vi "A 侧面 处理函数CCD4.vi"(7 "Image Name":string="I1", 8 "error in (no error)":errorcluster caption="错误输入（无错误）", 9 "相机选择":T2="cam0" caption="Session Out CCD3", 10 "New Image":T1, 11 "ParamsUI":T3={"IsNorImage"=TRUE, "Exposure Values"=100289, "ImagePath"=path "C:/Users/hedongpo/Desktop/514-hdp/Alignment Assemble System/Test Picture/B/3.bmp", "相机选择"="cam4"} caption="参数界面" {"Exposure Values" scale=0.0..200000.0}) -> (0 "error out":errorcluster caption="错误输出", 2 "Session Out":T2, 3 "Image out":T1(plugin-control), 4 "数值":dbl)   [LabVIEW 2017]
uses:
  <vilib>/userdefined/High Color/IMAQdx.ctl
  <vilib>/vision/Image Controls.llb/IMAQ Image.ctl
  <vilib>/vision/driver/IMAQdx.llb/IMAQdx Buffer Number Mode.ctl
  <resource>/objmgr/imaqdx.rc
  Global System.vi
  <vilib>/vision/driver/NI_Vision_Acquisition_Software.lvlib
  <vilib>/vision/NI_Vision_Development_Module.lvlib
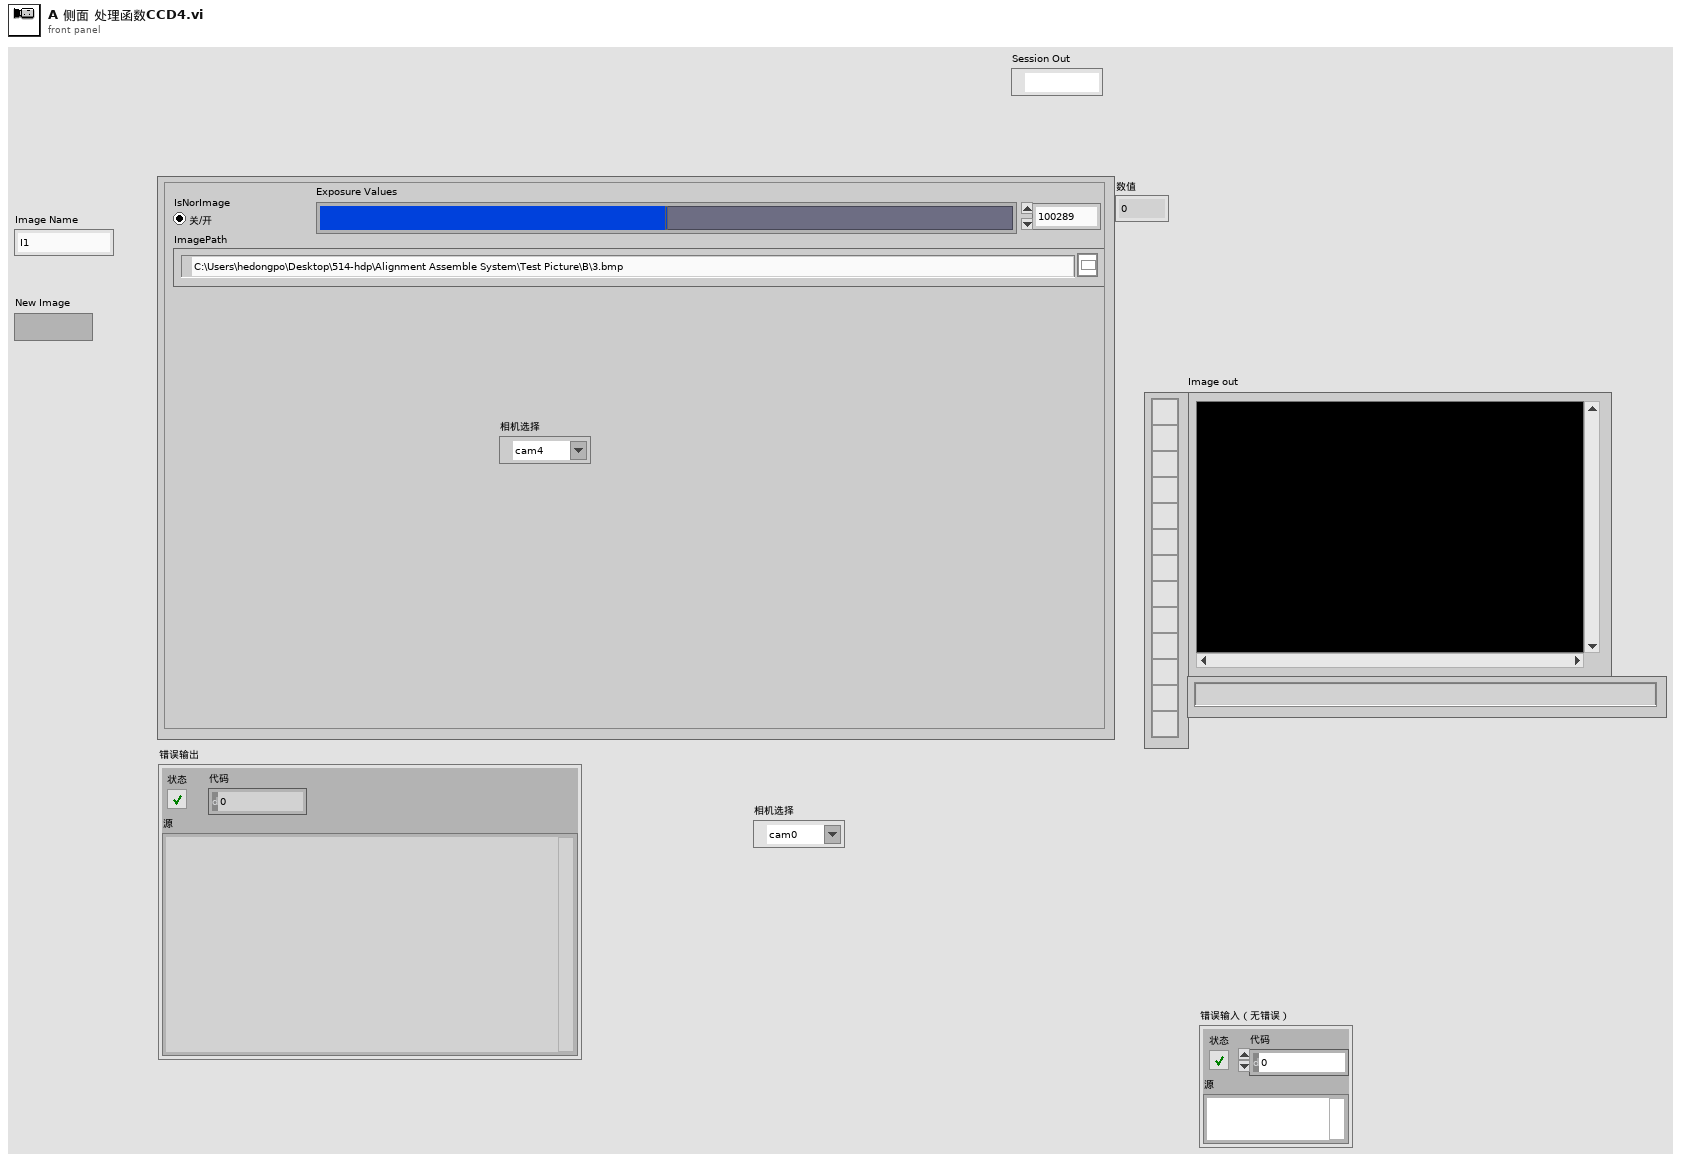
[diagram p1: front panel]
types:
  T1 = typedef "IMAQ Image.ctl" = refnum<image>
  T2 = typedef "IMAQdx.ctl" = refnum<k21>
  T3 = cluster{"IsNorImage":bool, "Exposure Values":i64, "ImagePath":path, "相机选择":T2}
  T4 = typedef "Image Type" = u32
  T5 = cluster{"IsNorImage":bool, "Exposure Values":u32, "ImagePath":path}
  T6 = typedef "NI_Vision_Acquisition_Software.lvlib/IMAQdx Buffer Number Mode.ctl" = enum32{"Next", "Last", "Buffer Number", "Every", "Last New"}
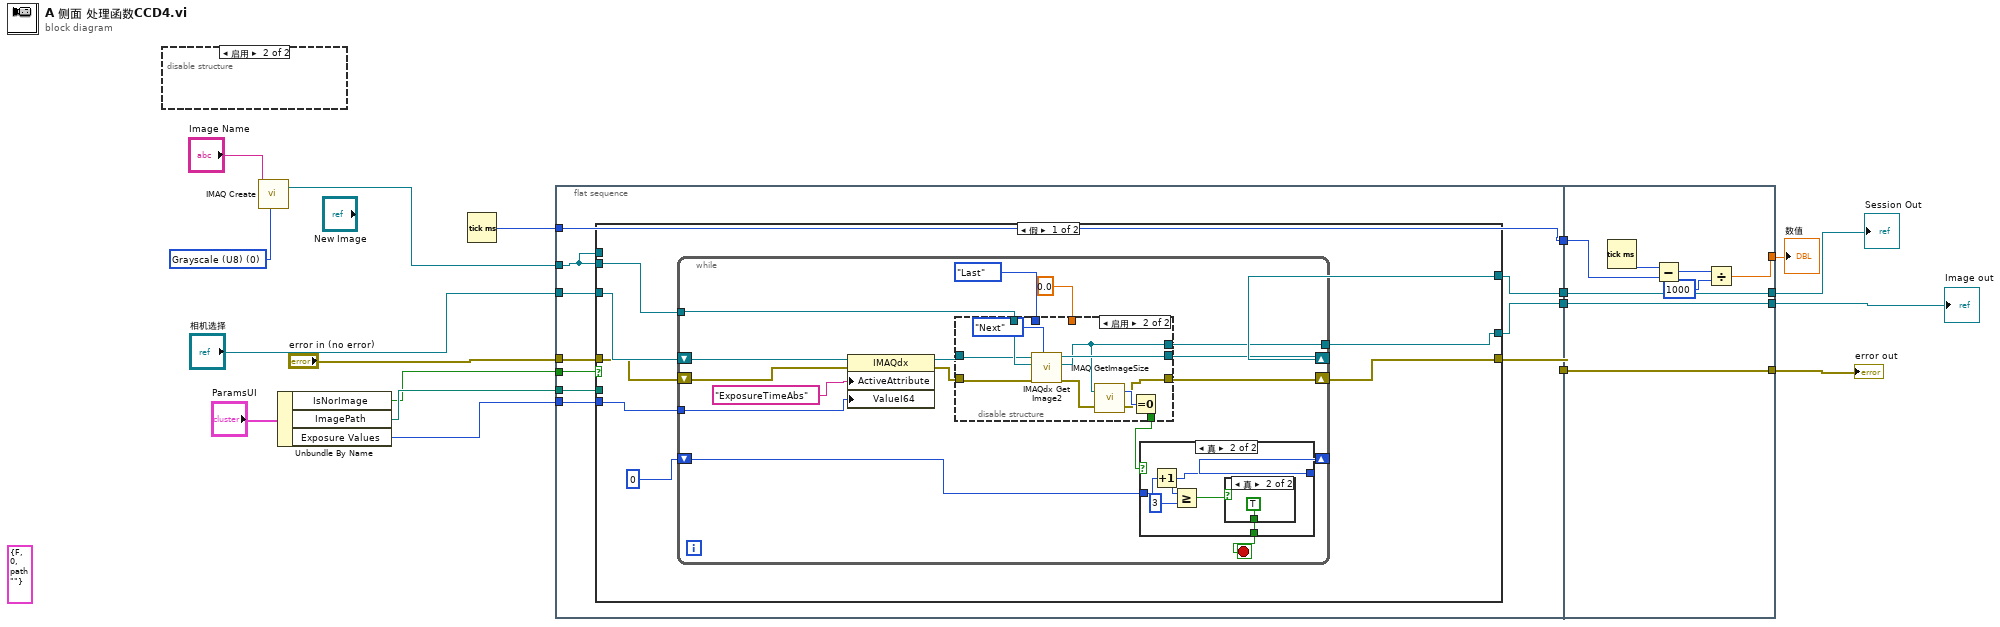
[diagram p0: block diagram]
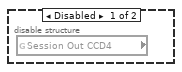
[diagram p2: hidden frame]
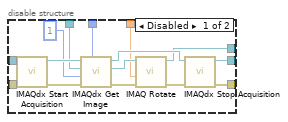
[diagram p3: hidden frame]
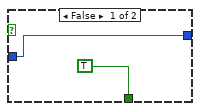
[diagram p4: hidden frame]
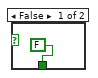
[diagram p5: hidden frame]
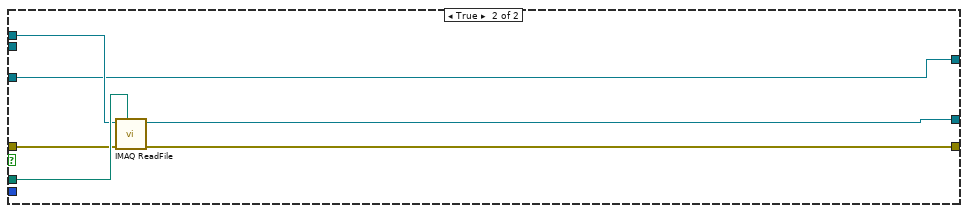
[diagram p6: hidden frame]
diagram:
  w2 = T4 0 items=["Grayscale (U8)", "Grayscale (I16)", "Grayscale (SGL)", "Complex (CSG)", "RGB (U32)", "HSL (U32)", "RGB (U64)", "Grayscale (U16)"] ("Image Type")
  (unwired) T5 {"IsNorImage"=FALSE, "Exposure Values"=0, "ImagePath"=path ""} ("ParamsUI")
  n1 = disable-structure shown="启用" {
    frame Disabled {
      n2 = global read "Global System.vi" "Session Out CCD4"() -> ()  [unwired: 1 out]
    }
    frame Enabled {
    }
  }
  n3 = call "IMAQ Create"("Image Name"="Image Name", "Image Type"=w2) -> ("New Image"=w1:T1)  [unwired: 3 in, 1 out]
  n4 = Unbundle By Name("ParamsUI") -> ("IsNorImage"=w5:bool, "ImagePath"=w6:path, "Exposure Values"=w18:i64)
  n5 = Tick Count (ms)() -> (millisecond timer value=w12:u32)
  n6 = flat-sequence {
    tunnel: w5 -> [w28]
    tunnel: w6 -> [w27]
    tunnel: w18 -> [w26]
    tunnel: w1 -> [w19]
    tunnel: "error in (no error)" -> [w25]
    tunnel: "相机选择" -> [w22]
    tunnel: w12 -> [w20]
    tunnel: [w24] -> w11
    tunnel: [w23] -> w10
    tunnel: [w21] -> w9
    tunnel: [w20] -> w8
    tunnel: [w98] -> w13
    tunnel: [w99] -> w14
    tunnel: [w100] -> w16
    tunnel: w11 -> [w100]
    tunnel: w10 -> [w99]
    tunnel: w9 -> [w98]
    tunnel: w8 -> [w96]
    tunnel: [w93] -> w7
    frame #0 {
      n7 = case shown="假" w28 {
        tunnel: w27 -> [_ w92]
        tunnel: [w29 w91] -> w23
        tunnel: w26 -> [w34 _]
        tunnel: w22 -> [w36 w87]
        tunnel: w19 -> [_ w90]
        tunnel: w25 -> [w35 w89]
        tunnel: [w30 w88] -> w24
        tunnel: [w31 w87] -> w21
        tunnel: w19 -> [w32 _]
        frame False {
          n8 = while {
            tunnel: w34 -> [w50]
            shift-right: [w39] -> w31
            shift-left: w36 -> [w52]
            shift-right: [w40] -> w30
            shift-left: w35 -> [w51]
            shift-right: [w47] -> _
            shift-left: 0 -> [w48]
            tunnel: w32 -> [w43]
            tunnel: [w38] -> w29
            stop <- w46 stop-if-true
            n9 = property class="IMAQdx"(reference=w52, error in=w51, "ActiveAttribute"="ExposureTimeAbs", "ValueI64"=w50) -> (reference out=w42:T2, error out=w41:errorcluster)
            n10 = disable-structure shown="启用" {
              disable-tunnel: IMAQdx_Buffer_Number_Mode."Last" ("Buffer Number Mode (Next)") -> [w64 _]
              disable-tunnel: sgl 0.0 ("Angle (degrees)") -> [w59 _]
              disable-tunnel: w43 -> [w58 w76]
              disable-tunnel: [w57 w73] -> w38
              disable-tunnel: [w56 w74] -> w39
              disable-tunnel: [w55 w69] -> w40
              disable-tunnel: w42 -> [w54 w75]
              disable-tunnel: w41 -> [w53 w77]
              disable-tunnel: [_ w71] -> w37
              frame Disabled {
                n11 = call <vilib>:"IMAQdx Start Acquisition.vi"("error in"=w53, "Session In"=w54) -> ("error out"=w66:errorcluster, "Session Out"=w67:T2)  [unwired: 8 in]
                n12 = call <vilib>:"IMAQdx Get Image.vi"("Buffer Number Mode (Next)"=w64, "error in"=w66, "Buffer Number In"=u32 1, "Image In"=w58, "Session In"=w67) -> ("error out"=w61:errorcluster, "Image Out"=w62:T1, "Session Out"=w63:T2)  [unwired: 3 in, 1 out]
                n13 = call "IMAQ Rotate"("error in (no error)"=w61, "Angle (degrees)"=w59, "Image Src"=w62) -> ("error out"=w60:errorcluster, "Image Dst Out"=w57:T1)  [unwired: 7 in]
                n14 = call <vilib>:"IMAQdx Stop Acquisition.vi"("error in"=w60, "Session In"=w63) -> ("error out"=w55:errorcluster, "Session Out"=w56:T2)  [unwired: 8 in]
              }
              frame Enabled {
                n15 = call <vilib>:"IMAQdx Get Image2.vi"("Buffer Number Mode (Next)"=IMAQdx_Buffer_Number_Mode."Next", "error in"=w77, "Image In"=w76, "Session In"=w75) -> ("error out"=w70:errorcluster, "Image Out"=w73:T1, "Session Out"=w74:T2)  [unwired: 4 in, 1 out]
                n16 = call "IMAQ GetImageSize"("Image"=w73, "error in (no error)"=w70) -> ("Y Resolution"=w72:i32, "error out"=w69:errorcluster)  [unwired: 2 in, 1 out]
                n17 = Equal To 0?(x=w72) -> (x = 0?=w71:bool)
              }
            }
            n18 = case shown="真" w37 {
              tunnel: w48 -> [w78 w84]
              tunnel: [w78 w81] -> w47
              tunnel: [TRUE w80] -> w46
              frame False {
              }
              frame True {
                n19 = Increment(x=w84) -> (x+1=w81:i32)
                n20 = Greater Or Equal?(x=w81, y=3) -> (x >= y?=w82:bool)
                n21 = case shown="真" w82 {
                  tunnel: [FALSE TRUE] -> w80
                  frame False {
                  }
                  frame True {
                  }
                }
              }
            }
          }
        }
        frame True {
          n22 = call "IMAQ ReadFile"("File Path"=w92, "error in (no error)"=w89, "Image"=w90) -> ("error out"=w88:errorcluster, "Image Out"=w91:T1)  [unwired: 4 in, 3 out]
        }
      }
    }
    frame #1 {
      n23 = Tick Count (ms)() -> (millisecond timer value=w97:u32)
      n24 = Subtract(x=w97, y=w96) -> (x-y=w95:u32)
      n25 = Divide(x=w95, y=u32 1000) -> (x/y=w93:dbl)
    }
  }
  "Image out" <- w14
  "error out" <- w16
  "Session Out" <- w13
  "数值" <- w7
